vi "2.2.vi"() -> ()   [LabVIEW 2020]
uses:
  <vilib>/numeric/Random Number (Range) I64.vi
  <vilib>/numeric/sub_Random U32.vi
panel:
  out "max value ºC":u64
  out "min index ºC":i32
  out "min index ºF, ºC, FILTRO":i32
  out "max value ºF, ºC, FILTRO":u64
  out "Array":dbl[][](array[numeric])
  out "Valores en °C":i64[](graph)
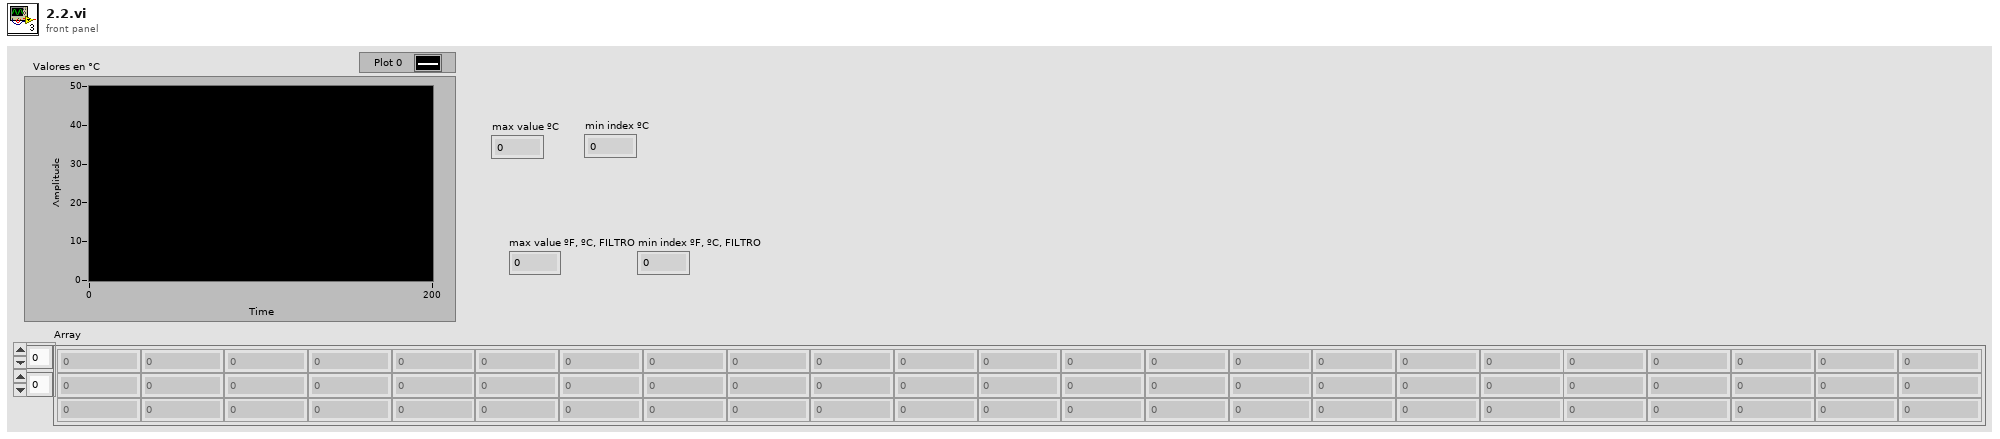
[diagram p1: front panel]
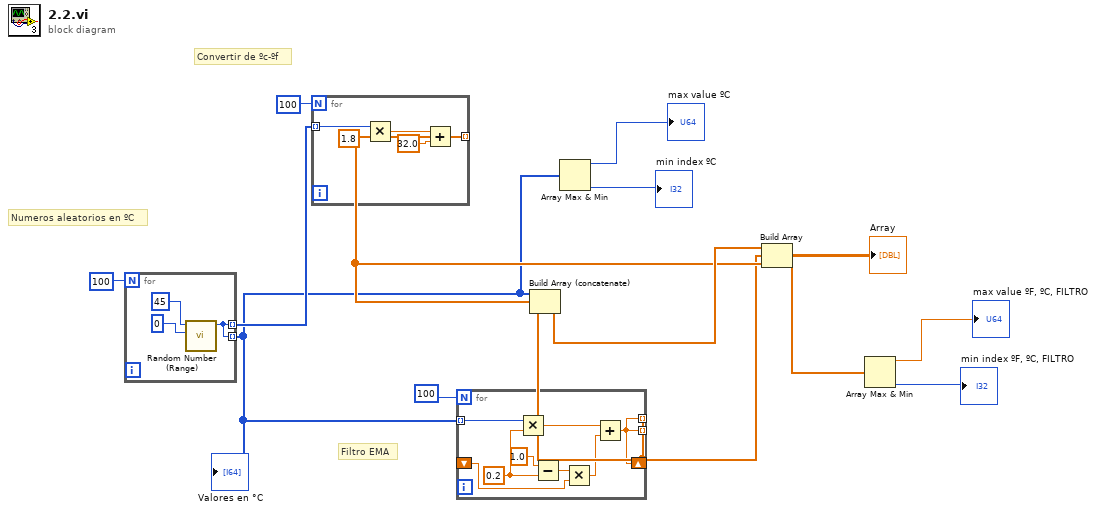
[diagram p0: block diagram]
diagram:
  # "Filtro EMA"
  # "Convertir de ºc-ºf"
  # "Numeros aleatorios en ºC"
  n1 = for {
    N: 100 -> [_]
    tunnel: [w15] -> w1 mode=indexing
    tunnel: [w15] -> w12 mode=indexing
    n2 = call-poly <vilib>:"Random Number (Range).vi"("lower bound (-100)"=u64 0 ("lower bound (0)"), "upper bound (100)"=u64 45) -> ("number"=w15:i64)  [unwired: 9 in]
  }
  "Valores en °C" <- w1
  n3 = for {
    N: 100 -> [_]
    tunnel: w12 -> [w18] mode=indexing
    tunnel: [w17] -> w5 mode=indexing
    n4 = Multiply(x=w18, y=1.8 ("x*y")) -> (x*y=w20:dbl)
    n5 = Add(x=w20, y=32.0) -> (x+y=w17:dbl)
  }
  n6 = for {
    N: 100 -> [_]
    tunnel: w1 -> [w29] mode=indexing
    shift-right: [w22] -> _
    shift-left: _ -> [w23]
    tunnel: [w22] -> _ mode=indexing
    tunnel: [w22] -> w4 mode=indexing
    w27 = 0.2 ("y")
    n7 = Multiply(x=w29, y=w27) -> (x*y=w25:dbl)
    n8 = Subtract(x=1.0, y=w27) -> (x-y=w26:dbl)
    n9 = Multiply(x=w26, y=w23) -> (x*y=w24:dbl)
    n10 = Add(x=w25, y=w24) -> (x+y=w22:dbl)
  }
  n11 = Build Array (concatenate) "Build Array"(w1, w5, w4) -> (w6:dbl[])
  n12 = Array Max & Min(array=w1) -> (max value=→"max value ºC":i64, min index (indices)=→"min index ºC":i32)  [unwired: 2 out]
  n13 = Build Array(w6, w4, w5) -> (→"Array":dbl[][])
  n14 = Array Max & Min(array=w6) -> (max value=→"max value ºF, ºC, FILTRO":dbl, min index (indices)=→"min index ºF, ºC, FILTRO":i32)  [unwired: 2 out]
